vi "基础21.vi"() -> ()   [LabVIEW 2014]
uses:
  <vilib>/Utility/file.llb/Write To Spreadsheet File (DBL).vi
panel:
  in  "停止":bool
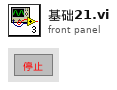
[diagram p1: front panel]
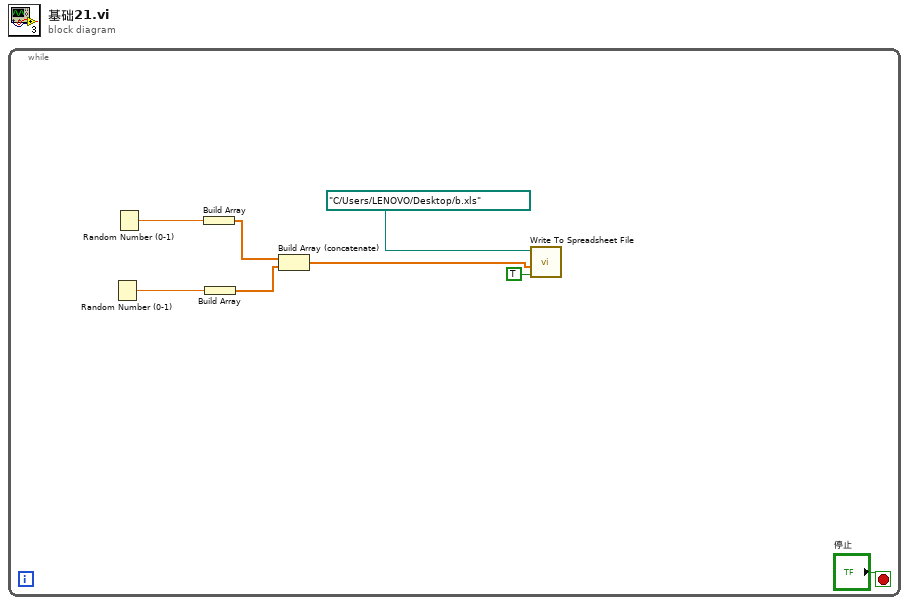
[diagram p0: block diagram]
diagram:
  n1 = while {
    stop <- "停止" stop-if-true
    n2 = Random Number (0-1)() -> (number: 0 to 1=w5:dbl)
    n3 = Random Number (0-1)() -> (number: 0 to 1=w6:dbl)
    n4 = Build Array(w6) -> (w4:dbl[])
    n5 = Build Array(w5) -> (w3:dbl[])
    n6 = Build Array (concatenate)(w4, w3) -> (w1:dbl[])
    n7 = call-poly <vilib>:"Write To Spreadsheet File.vi"("append to file? (new file:F)"=TRUE, "1D data"=w1, "file path (dialog if empty)"=path "C:/Users/LENOVO/Desktop/b.xls") -> ()  [unwired: 5 in, 1 out]
  }
